vi "Get Result.vi"(6 "Last request":bool, 8 "error in (no error)":errorcluster, 11 "Instrument Recorder in":refnum<class "Line Detector.lvclass">) -> (0 "error out":errorcluster, 2 "Result":refnum<class "Acquired Result.lvclass">, 3 "Instrument Recorder out":refnum<class "Line Detector.lvclass">)   [LabVIEW 2016, in "Line Detector.lvclass"]
uses:
  Line Detector.lvclass
  Results/Acquired Result/Acquired Result.lvclass
  Line Detector.lvclass/Line Detector.ctl
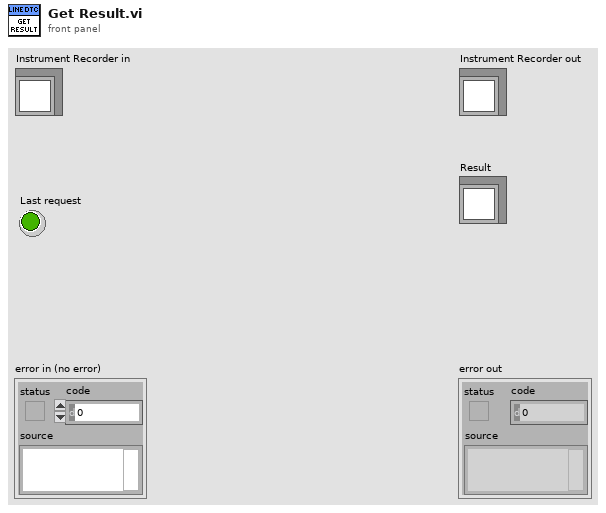
[diagram p1: front panel]
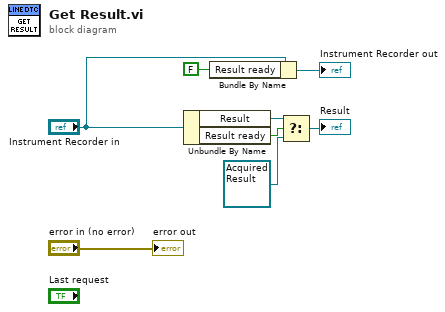
[diagram p0: block diagram]
diagram:
  n1 = Unbundle By Name("Instrument Recorder in") -> ("Result"=w7:refnum<class "Acquired Result.lvclass">, "Result ready"=w8:bool)
  n2 = Bundle By Name(cluster="Instrument Recorder in", "Result ready"=FALSE) -> (→"Instrument Recorder out":refnum<class "Line Detector.lvclass">)
  n3 = Select(t=w7, s=w8, f=refnum<class "Acquired Result.lvclass"> refnum) -> (s? t:f=→"Result":refnum<class "Acquired Result.lvclass">)
  "error out" <- "error in (no error)"
